vi "AutoKal GT Konzentration Filtern.vi"(9 "Index":i32, 10 "CG für KAL":T1[](array[typedef]), 11 "MB für KAL":u16[](array[numeric])) -> (0 "CG für KAL":T1, 1 "Messberich":T2, 2 "Konzentration":dbl, 3 "Fehler/Leer":bool)   [LabVIEW 2020, in "Auto Kalibrieren.lvlib"]
uses:
  Auto Kalibrieren.lvlib
  Seiten/CalGas Aufschaltung/Definition CalGas Anzeige.ctl
  Seiten/CalGas Aufschaltung/CalGas-Namen.ctl
  Visualisierungs Elemente/String - Eingabefeld.ctl
  Seiten/CalGas Aufschaltung/CalGas-Werte.ctl
  Visualisierungs Elemente/Zahlen-Eingabefeld.ctl
  Seiten/CalGas Aufschaltung/CalGas-Einheit.ctl
  Visualisierungs Elemente/Auswahlfeld.ctl
  Seiten/CalGas Aufschaltung/CalGas-Messbereiche.ctl
  Visualisierungs Elemente/String - Ausgabefeld.ctl
  Linearisierung V2/Aktion Lin Daten aufarbeiten.ctl
  Linearisierung V2/Linearisierung v2.lvlib
  Seiten/CalGas Aufschaltung/CalGas Aufschaltung.lvlib
panel:
  in  "Def.CalGas":T3 {"Messbereiche"."Messbereich 12" items=["0-100ppm", "0-1000ppm", "0-5000ppm"]; "Messbereiche"."Messbereich 11" items=["0-100ppm", "0-1000ppm", "0-5000ppm"]; "Messbereiche"."Messbereich 10" items=["0-100ppm", "0-1000ppm", "0-5000ppm"]; "Messbereiche"."Messbereich 9" items=["0-100ppm", "0-1000ppm", "0-5000ppm"]; "Messbereiche"."Messbereich 8" items=["0-100ppm", "0-1000ppm", "0-5000ppm"]; "Messbereiche"."Messbereich 7" items=["0-100ppm", "0-1000ppm", "0-5000ppm"]; "Messbereiche"."Messbereich 6" items=["0-100ppm", "0-1000ppm", "0-5000ppm"]; "Messbereiche"."Messbereich 5" items=["0-100ppm", "0-1000ppm", "0-5000ppm"]; "Messbereiche"."Messbereich 4" items=["0-100ppm", "0-1000ppm", "0-5000ppm"]; "Messbereiche"."Messbereich 3" items=["0-100ppm", "0-1000ppm", "0-5000ppm"]; "Messbereiche"."Messbereich 2" items=["0-100ppm", "0-1000ppm", "0-5000ppm"]; "Messbereiche"."Messbereich 1" items=["0-100ppm", "0-1000ppm", "0-5000ppm"]; "Einheit"."Einheit 12" items=["ppm", "%"]; "Einheit"."Einheit 11" items=["ppm", "%"]; "Einheit"."Einheit 10" items=["ppm", "%"]; "Einheit"."Einheit 9" items=["ppm", "%"]; "Einheit"."Einheit 8" items=["ppm", "%"]; "Einheit"."Einheit 7" items=["ppm", "%"]; "Einheit"."Einheit 6" items=["ppm", "%"]; "Einheit"."Einheit 5" items=["ppm", "%"]; "Einheit"."Einheit 4" items=["ppm", "%"]; "Einheit"."Einheit 3" items=["ppm", "%"]; "Einheit"."Einheit 2" items=["ppm", "%"]; "Einheit"."Einheit 1" items=["ppm", "%"]; "Werte 2"."Konzentration 12" format="%#_5g"; "Werte 2"."Konzentration 11" format="%#_5g"; "Werte 2"."Konzentration 10" format="%#_5g"; "Werte 2"."Konzentration 9" format="%#_5g"; "Werte 2"."Konzentration 8" format="%#_5g"; "Werte 2"."Konzentration 7" format="%#_5g"; "Werte 2"."Konzentration 6" format="%#_5g"; "Werte 2"."Konzentration 5" format="%#_5g"; "Werte 2"."Konzentration 4" format="%#_5g"; "Werte 2"."Konzentration 3" format="%#_5g"; "Werte 2"."Konzentration 2" format="%#_5g"; "Werte 2"."Konzentration 1" format="%#_5g"; "Werte"."Konzentration 12" format="%#_5g"; "Werte"."Konzentration 11" format="%#_5g"; "Werte"."Konzentration 10" format="%#_5g"; "Werte"."Konzentration 9" format="%#_5g"; "Werte"."Konzentration 8" format="%#_5g"; "Werte"."Konzentration 7" format="%#_5g"; "Werte"."Konzentration 6" format="%#_5g"; "Werte"."Konzentration 5" format="%#_5g"; "Werte"."Konzentration 4" format="%#_5g"; "Werte"."Konzentration 3" format="%#_5g"; "Werte"."Konzentration 2" format="%#_5g"; "Werte"."Konzentration 1" format="%#_5g"}
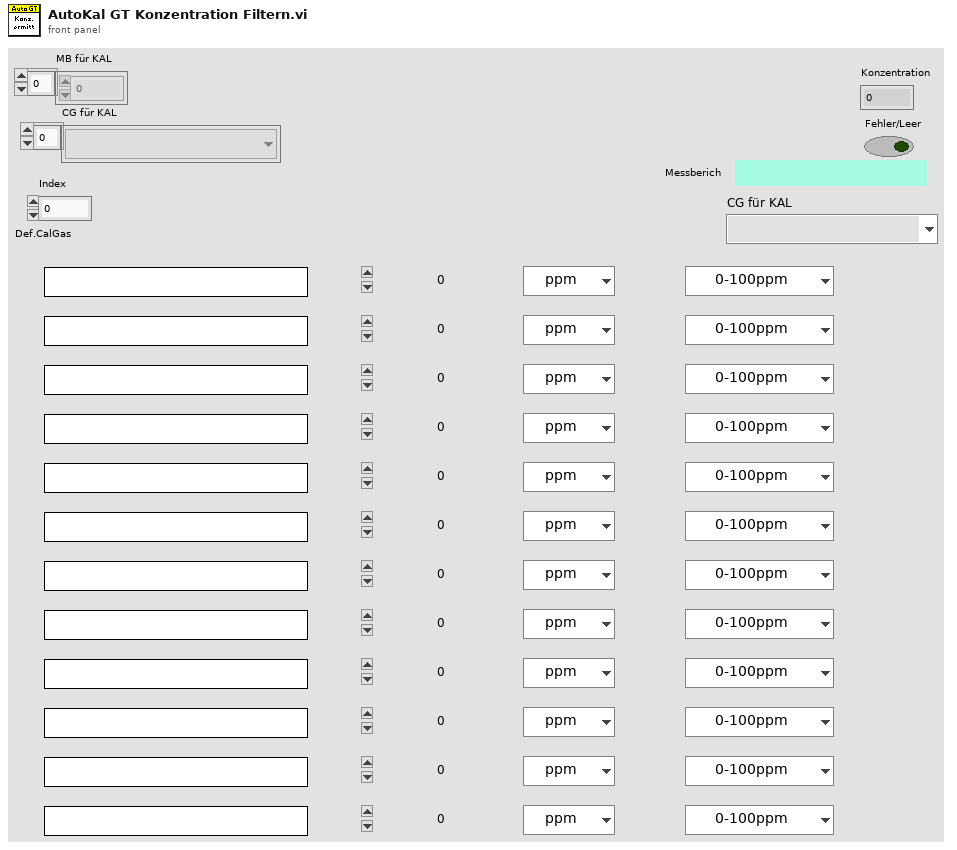
[diagram p1: front panel]
types:
  T1 = typedef "Auswahlfeld.ctl" = u16
  T2 = typedef "String - Ausgabefeld.ctl" = string
  T3 = typedef "CalGas Aufschaltung.lvlib/Definition CalGas Anzeige.ctl" = cluster{"Namen":T4, "Werte":T6, "Werte 2":T6, "Einheit":T8, "Messbereiche":T9}
  T4 = typedef "CalGas Aufschaltung.lvlib/CalGas-Namen.ctl" = cluster{"Name":T5, "Name 2":T5, "Name 3":T5, "Name 4":T5, "Name 5":T5, "Name 6":T5, "Name 7":T5, "Name 8":T5, "Name 9":T5, "Name 10":T5, "Name 11":T5, "Name 12":T5}
  T5 = typedef "String - Eingabefeld.ctl" = string
  T6 = typedef "CalGas Aufschaltung.lvlib/CalGas-Werte.ctl" = cluster{"Konzentration 1":T7, "Konzentration 2":T7, "Konzentration 3":T7, "Konzentration 4":T7, "Konzentration 5":T7, "Konzentration 6":T7, "Konzentration 7":T7, "Konzentration 8":T7, "Konzentration 9":T7, "Konzentration 10":T7, "Konzentration 11":T7, "Konzentration 12":T7}
  T7 = typedef "Zahlen-Eingabefeld.ctl" = sgl
  T8 = typedef "CalGas Aufschaltung.lvlib/CalGas-Einheit.ctl" = cluster{"Einheit 1":T1, "Einheit 2":T1, "Einheit 3":T1, "Einheit 4":T1, "Einheit 5":T1, "Einheit 6":T1, "Einheit 7":T1, "Einheit 8":T1, "Einheit 9":T1, "Einheit 10":T1, "Einheit 11":T1, "Einheit 12":T1}
  T9 = typedef "CalGas Aufschaltung.lvlib/CalGas-Messbereiche.ctl" = cluster{"Messbereich 1":T1, "Messbereich 2":T1, "Messbereich 3":T1, "Messbereich 4":T1, "Messbereich 5":T1, "Messbereich 6":T1, "Messbereich 7":T1, "Messbereich 8":T1, "Messbereich 9":T1, "Messbereich 10":T1, "Messbereich 11":T1, "Messbereich 12":T1}
  T10 = typedef "Linearisierung v2.lvlib/Aktion Lin Daten aufarbeiten.ctl" = enum16{"lesen", "Protkolldaten", "speichern", "laden", "EPA auswerten", "Tabelle schreiben", "Lin auswerten", "Tab init", "Stufentabelle", "EPA aktiviert", "Nachbehandlung laden", "Tabelle löschen", "Istwerte löschen", "Zeile löschen", "Zeile einfügen", "LIN aktiviert", "LIN/EPA aktiv laden", "EGAK Tab", "LIN übernehmen", "Tab init ohne Stufen"}
  T11 = typedef "Linearisierung v2.lvlib/Lin-Polynom Daten.ctl" = cluster{"Messgerät":string, "Kalibrator (Gasteiler)":string, "Bearbeiter/in":string, "Komponente":string, "Zeitstempel":timestamp, "F_max gefordert (%)":sgl, "F_max in %":sgl, "F_max in ppm":sgl, "Vorschlag Ordnung":i32, "Polynom OK":bool, "Polynomkoeff.":dbl[], "Prüfgas Konzentration":dbl, "Pfad EPA":string, "Pfad_LIN":string, "Gasnummer:":u8, "Komponentenauswahl":T12, "Verdünnungsgas":T13, "Zeitdauer Stufe":T7, "Anzahl Stufen":T7, "F_max in % EPA":sgl, "F_max in ppm EPA":sgl, "F_max in % LIN":sgl, "F_max in ppm LIN":sgl, "Punkte umkehren":bool, "EPA Optionsfeld":T14, "Autolin Hovacal":T15, "Spanfactors":sgl[], "Kalibrierauswahl":T16, "Conditions:":T17, "Gasflaschen Nr.:":string, "Bottle Accuracy":dbl, "Konfig Gasflasche":T18, "Gasflasche":T19, "HovaCAL Flow AutoLin":T20, "MFC Output":T21, "Gas Ablaufdatum":timestamp, "Lin Modus":T22, "zusätzliche Zeitdauer Erster Punkt":sgl, "Offsets":sgl[]}
  T12 = typedef "Linearisierung v2.lvlib/KomponentenArray.ctl" = cluster{"Komponente:":T1, "Konzentration":dbl}[]
  T13 = typedef "Linearisierung v2.lvlib/Gasteiler.lvlib/Prüfgas in.ctl" = u16
  T14 = typedef "Linearisierung v2.lvlib/EPA Optionsfeld.ctl" = enum32{"Istwert", "Rohwert", "Linearisierter Wert"}
  T15 = typedef "Linearisierung v2.lvlib/Gasteiler.lvlib/HovaCal.lvlib/AutoLin Hovacal.ctl" = enum32{"Keine Auswahl", "Optionsauswahl 1", "Optionsauswahl 2"}
  T16 = typedef "Linearisierung v2.lvlib/Kalibrieroption.ctl" = u16
  T17 = typedef "Linearisierung v2.lvlib/Linearity verification 1065-307.lvlib/Condition.ctl" = u16
  T18 = typedef "System Einstellungen V2.lvlib/Konfig Gasflasche.ctl" = bool
  T19 = typedef "System Einstellungen V2.lvlib/Gasflasche Auswahl.ctl" = u16
  T20 = typedef "Linearisierung v2.lvlib/Gasteiler.lvlib/HovaCAL_Interface.lvlib/Controls.lvlib/Flow Einstellung.ctl" = cluster{"HovaCAL Flow Input Cluster":dbl}
  T21 = typedef "Linearisierung v2.lvlib/Gasteiler.lvlib/HovaCAL_Interface.lvlib/Controls.lvlib/Pump state.ctl" = cluster{"Run":bool}
  T22 = typedef "CalGas Aufschaltung.lvlib/Lin Modus.ctl" = u16
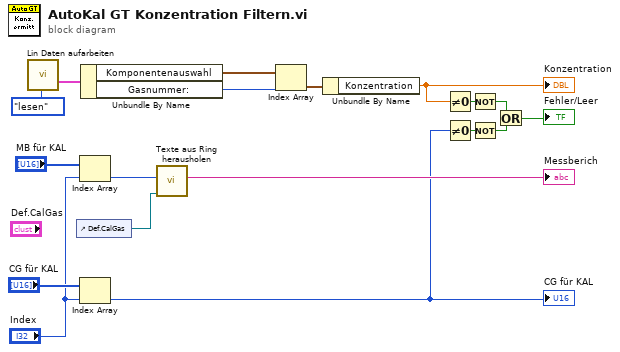
[diagram p0: block diagram]
diagram:
  n1 = call "Lin Daten aufarbeiten.vi"("Aktionen"=Aktion_Lin_Daten_aufarbeiten."lesen") -> ("Lin-Polynom"=w15:T11)  [unwired: 16 in, 10 out]
  n2 = control-ref of="Def.CalGas"() -> (w9:refnum<vi>)
  n3 = Index Array(array="MB für KAL", index="Index") -> (element=w10:u16)
  n4 = Index Array(array="CG für KAL", index="Index") -> (element=w5:T1)
  "CG für KAL" <- w5
  n5 = Unbundle By Name(w15) -> ("Komponentenauswahl"=w14:T12, "Gasnummer:"=w13:u8)
  n6 = call "Texte aus Ring herausholen.vi"("Def.CalGas"=w9, "Element Messbereich"=w10) -> ("Messberich"=→"Messberich":T2)  [unwired: 8 in, 1 out]
  n7 = Index Array(array=w14, index=w13) -> (element=w12:cluster{"Komponente:":T1, "Konzentration":dbl})
  n8 = Unbundle By Name(w12) -> ("Konzentration"=w17:dbl)
  "Konzentration" <- w17
  n9 = Not Equal To 0?(x=w17) -> (x != 0?=w18:bool)
  n10 = Not Equal To 0?(x=w5) -> (x != 0?=w1:bool)
  n11 = Not(x=w18) -> (.not. x?=w4:bool)
  n12 = Not(x=w1) -> (.not. x?=w3:bool)
  n13 = Or(x=w4, y=w3) -> (x .or. y?=→"Fehler/Leer":bool)
